vi "Is Initialized.vi"(8 "error in":errorcluster, 11 "Virtual Sensor from CSV in":refnum<class "Virtual Sensor from CSV.lvclass">) -> (0 "error out":errorcluster, 2 "Is Initialized?":bool, 3 "Virtual Sensor from CSV out":refnum<class "Virtual Sensor from CSV.lvclass">)   [LabVIEW 2024, in "Virtual Sensor from CSV.lvclass"]
uses:
  Virtual Sensor from CSV.lvclass
  Virtual Sensor from CSV.lvclass/Virtual Sensor from CSV.ctl
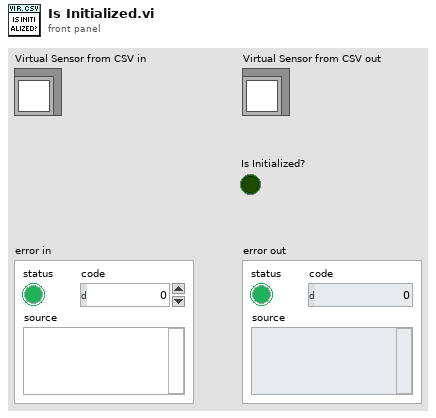
[diagram p1: front panel]
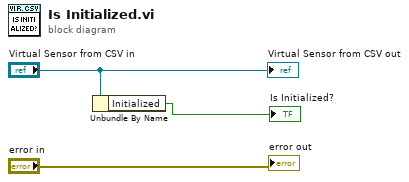
[diagram p0: block diagram]
diagram:
  n1 = Unbundle By Name("Virtual Sensor from CSV in") -> ("Initialized"=→"Is Initialized?":bool)
  "Virtual Sensor from CSV out" <- "Virtual Sensor from CSV in"
  "error out" <- "error in"
